vi "PH_Beckhoff_PPMA-Rods.set i Attr and open Services.vi"(2 "error in":errorcluster) -> (0 "error out":errorcluster, 1 "i Attr":T1 {"States"."Status" items=["no info", "off/false/out", "on/true/in", "Failure", "Alarm", "Status 1", "Status 2", "Status 3"]})   [LabVIEW 2014, in "PH_Beckhoff_PPMA-Rods.lvlib"]
uses:
  PH_Beckhoff_PPMA-Rods.lvlib
  PH_Beckhoff_PPMA-Rods.i attribute.ctl
  PH_StatusHandler/PH_StatusHandler.GUI element.ctl
  PH_StatusHandler/PH_StatusHandler.Status.ctl
  PH_Beckhoff_PPMA-Rods.Rods Tags.ctl
  lib.lib/DimLVEvent/LVDimInterface/LVDimInterface.lvlib
  PH_StatusHandler/PH_StatusHandler.lvlib
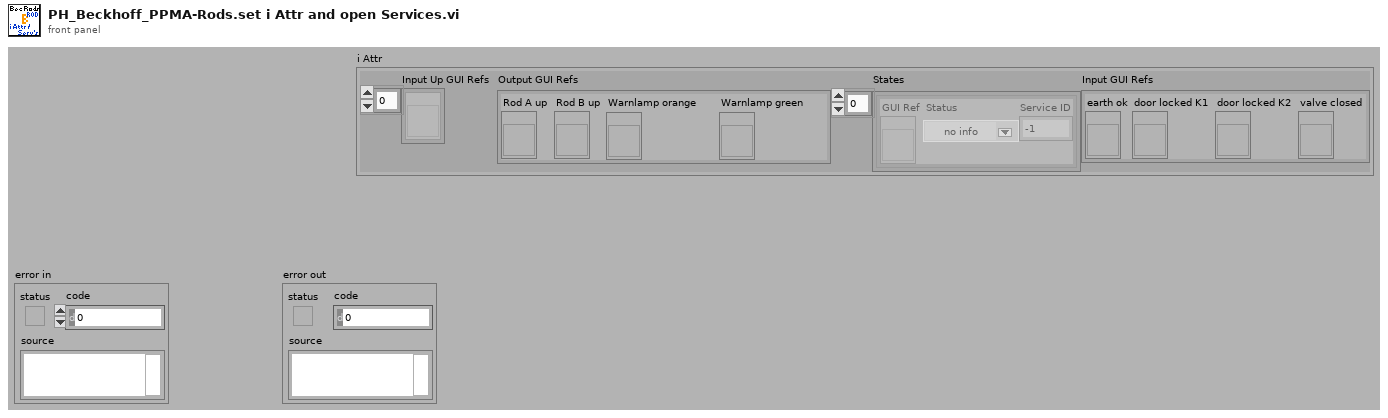
[diagram p1: front panel]
types:
  T1 = typedef "PH_Beckhoff_PPMA-Rods.lvlib/PH_Beckhoff_PPMA-Rods.i attribute.ctl" = cluster{"Input Up GUI Refs":refnum<vi>[], "Output GUI Refs":cluster{"Rod A up":refnum<vi>, "Rod B up":refnum<vi>, "Warnlamp orange":refnum<vi>, "Warnlamp green":refnum<vi>}, "States":cluster{"GUI Ref":refnum<vi>, "Status":T2, "Service ID":i32}[], "Input GUI Refs":cluster{"earth ok":refnum<vi>, "door locked K1":refnum<vi>, "door locked K2":refnum<vi>, "valve closed":refnum<vi>}}
  T2 = typedef "PH_StatusHandler.lvlib/PH_StatusHandler.Status.ctl" = i16
  T3 = cluster{"GUI Ref":refnum<vi>, "Status":T2, "Service ID":i32}
  T4 = typedef "PH_Beckhoff_PPMA-Rods.lvlib/PH_Beckhoff_PPMA-Rods.Rods Tags.ctl" = enum16{"Rod-up", "earth-ok", "door-locked-K1", "door-locked-K2", "watervalve-closed", "Rods-Chain-A-up", "Rods-Chain-B-up", "HV-Warnlamp-orange", "HV-Warnlamp-green", "Status-Rods-PU-1", "Status-Rods-PU-2", "Status-Rods-PU-3", "Status-Rods-PU-4", "Status-Rods-PU-5", "Status-Rods-PU-6", "Status-Rods-PU-7", "Status-Rods-PU-8", "Status-Rods-PU-9", "Status-Rods-PU-10", "Status-Rods-FR", "Status-Rods-PILC"}
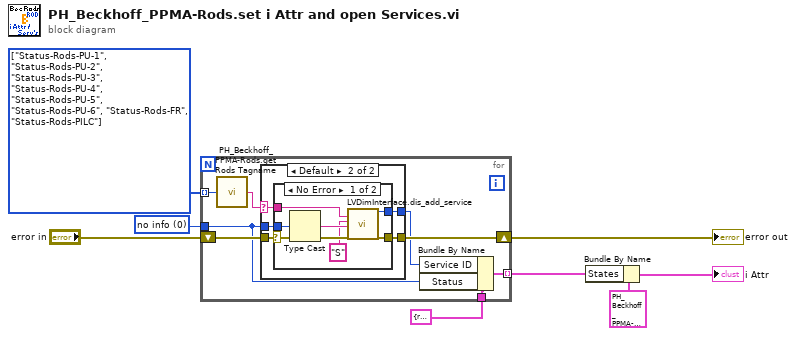
[diagram p0: block diagram]
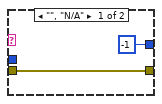
[diagram p2: hidden frame]
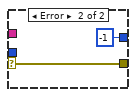
[diagram p3: hidden frame]
diagram:
  w5 = T4[] [enum."Status-Rods-PU-1", enum."Status-Rods-PU-2", enum."Status-Rods-PU-3", enum."Status-Rods-PU-4", enum."Status-Rods-PU-5", enum."Status-Rods-PU-6", enum."Status-Rods-FR", enum."Status-Rods-PILC"] items=["Rod-up", "earth-ok", "door-locked-K1", "door-locked-K2", "watervalve-closed", "Rods-Chain-A-up", "Rods-Chain-B-up", "HV-Warnlamp-orange", "HV-Warnlamp-green", "Status-Rods-PU-1", "Status-Rods-PU-2", "Status-Rods-PU-3", "Status-Rods-PU-4", "Status-Rods-PU-5", "Status-Rods-PU-6", "Status-Rods-PU-7", "Status-Rods-PU-8", "Status-Rods-PU-9", "Status-Rods-PU-10", "Status-Rods-FR", "Status-Rods-PILC"]
  w6 = T2 0 items=["no info", "off/false/out", "on/true/in", "Failure", "Alarm", "Status 1", "Status 2", "Status 3"] ("Status")
  n1 = for {
    shift-right: [w13] -> w8
    shift-left: "error in" -> [w14]
    tunnel: [w16] -> w2 mode=indexing
    tunnel: T3 {"GUI Ref"=refnum, "Status"=0, "Service ID"=0} ("PSU Data") -> [w15]
    tunnel: w6 -> [w12]
    tunnel: w5 -> [w9] mode=indexing
    n2 = call "PH_Beckhoff_PPMA-Rods.get Rods Tagname.vi"("Rods Tag"=w9) -> ("Rods Tagname"=w11:string)
    n3 = case shown="Default" w11 {
      selector: w11 -> [_ w19]
      tunnel: w14 -> [w18 w23]
      tunnel: [w18 w22] -> w13
      tunnel: [-1 ("my_serviceID") w21] -> w10
      tunnel: w12 -> [_ w20]
      frame "", "N/A" {
      }
      frame Default {
        n4 = case shown="No Error" w23 {
          selector: w23 -> [w28 w32]
          tunnel: [w30 -1 ("my_serviceID")] -> w21
          tunnel: [w29 w32] -> w22
          tunnel: w20 -> [w27 _]
          tunnel: w19 -> [w24 _]
          frame No Error {
            n5 = Type Cast(x=w27) -> (*(type *) &x=w26:string)  [unwired: 1 in]
            n6 = call "LVDimInterface.dis_add_service.vi"("serviceName"=w24, "typeDescriptor"="S", "data"=w26, "error in (no error)"=w28) -> ("my_serviceID"=w30:i32, "error out"=w29:errorcluster)  [unwired: 14 in]
          }
          frame Error {
          }
        }
      }
    }
    n7 = Bundle By Name(cluster=w15, "Service ID"=w10, "Status"=w12) -> (w16:T3)
  }
  "error out" <- w8
  n8 = Bundle By Name(cluster=T1 {"Input Up GUI Refs"=[], "Output GUI Refs"={"Rod A up"=refnum, "Rod B up"=refnum, "Warnlamp orange"=refnum, "Warnlamp green"=refnum}, "States"=[], "Input GUI Refs"={"earth ok"=refnum, "door locked K1"=refnum, "door locked K2"=refnum, "valve closed"=refnum}} ("i Attr"), "States"=w2) -> (→"i Attr":T1)
